vi "Display WebPubURL.vi"(8 "error in (no error)":errorcluster, 11 "CS++BaseActor in":refnum<class "CS++BaseActor.lvclass">) -> (0 "error out":errorcluster, 3 "CS++BaseActor out":refnum<class "CS++BaseActor.lvclass">)   [LabVIEW 2016, in "CS++BaseActor.lvlib" / "CS++BaseActor.lvclass"]
doc: "Display Web-Publishing URL in modal Dialog."
uses:
  CS++BaseActor.lvclass
  CS++BaseActor.lvclass/CS++BaseActor.ctl
panel:
  out "WebPub.Enabled":bool
  in  "OK Button":bool
  out "WebPub.URL":string
  out "VI Clone Name":string
  out "Object Name":string
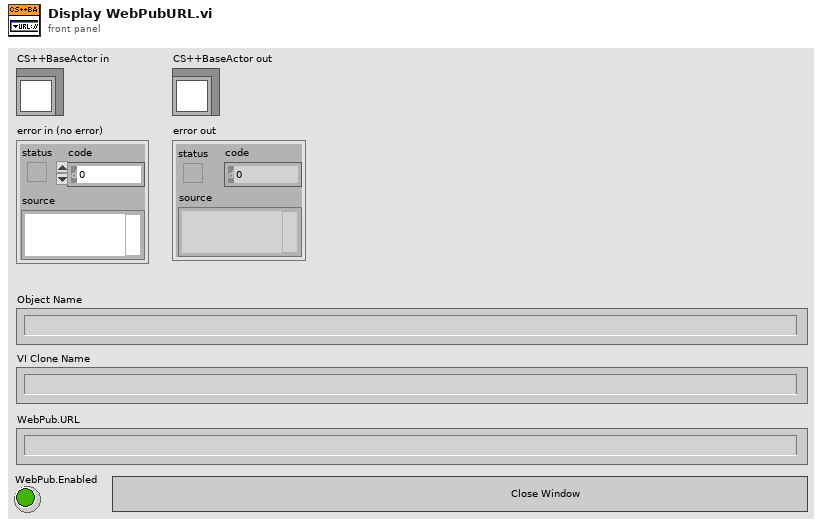
[diagram p1: front panel]
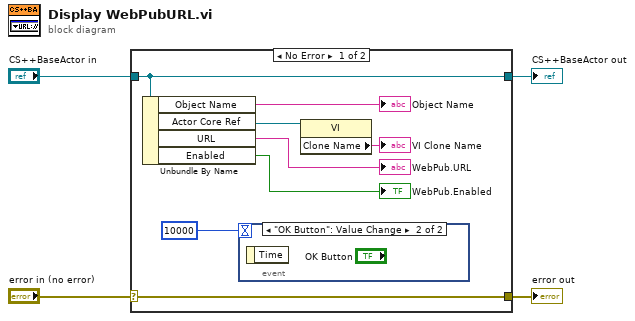
[diagram p0: block diagram]
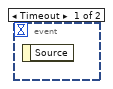
[diagram p2: hidden frame]
diagram:
  n1 = case shown="No Error" "error in (no error)" {
    selector: "error in (no error)" -> [w12 w14]
    tunnel: [w12 w14] -> w3
    tunnel: [w11 w13] -> w1
    tunnel: "CS++BaseActor in" -> [w11 w13]
    frame No Error {
      n2 = Unbundle By Name(w11) -> ("Object Name"=→"Object Name":string, "Actor Core Ref"=w10:refnum<vi>, "URL"=→"WebPub.URL":string, "Enabled"=→"WebPub.Enabled":bool)
      n3 = event shown="[1] \"OK Button\": Value Change" {
        selector: _ -> [_ _]
        dyn-events: _ -> [_ _]
        timeout: 10000 -> [_ _]
        event Timeout {
          n4 = event-data() -> ()  [unwired: 1 in, 1 out]
        }
        event "OK Button": Value Change {
          n5 = event-data() -> ()  [unwired: 1 in, 1 out]
        }
      }
      n6 = property class="VI"(reference=w10) -> ("Clone Name"=→"VI Clone Name":string)  [unwired: 1 in, 2 out]
    }
    frame Error {
    }
  }
  "error out" <- w3
  "CS++BaseActor out" <- w1
